vi "JoystickRotationScaling.vi"(2 "Rotation Scaling":dbl, 3 "Rotation Deadband":dbl, 4 "Raw Rotation Joystick":dbl) -> (0 "Scaled Rotation Joystick":dbl, 1 "Out of Deadband":bool)   [LabVIEW 2019]
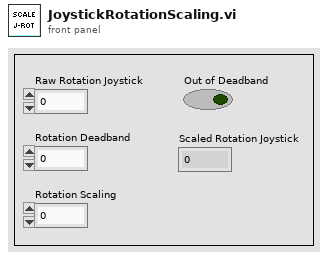
[diagram p1: front panel]
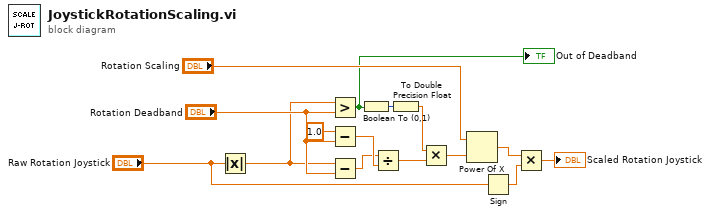
[diagram p0: block diagram]
diagram:
  n1 = Absolute Value(x="Raw Rotation Joystick") -> (abs(x)=w9:dbl)
  n2 = Greater?(x=w9, y="Rotation Deadband") -> (0:w10:bool)
  "Out of Deadband" <- w10
  n3 = Subtract(x=1.0, y="Rotation Deadband") -> (x-y=w5:dbl)
  n4 = Subtract(x=w9, y="Rotation Deadband") -> (x-y=w3:dbl)
  n5 = Boolean To (0,1)(Boolean=w10) -> (0, 1=w1:i16)
  n6 = Divide(x=w3, y=w5) -> (x/y=w6:dbl)
  n7 = To Double Precision Float(number=w1) -> (double precision float=w2:dbl)
  n8 = Multiply(x=w2, y=w6) -> (x*y=w13:dbl)
  n9 = Power Of X(1:w13, 2:"Rotation Scaling") -> (0:w14:dbl)
  n10 = Sign(1:"Raw Rotation Joystick") -> (0:w8:dbl)
  n11 = Multiply(x=w14, y=w8) -> (x*y=→"Scaled Rotation Joystick":dbl)
